vi "SetStringArray.vi"(4 "Sequence Context":T1) -> (0 "error out":errorcluster, 1 "Test Data":T2 {"Numeric Measurement" format="%.2f"})   [LabVIEW 2013]
uses:
  <vilib>/addons/TestStand/_TSLegacy.llb/LabVIEW Test - Test Data.ctl
  <vilib>/addons/TestStand/_TSLegacy.llb/LabVIEW Test - Sequence Context.ctl
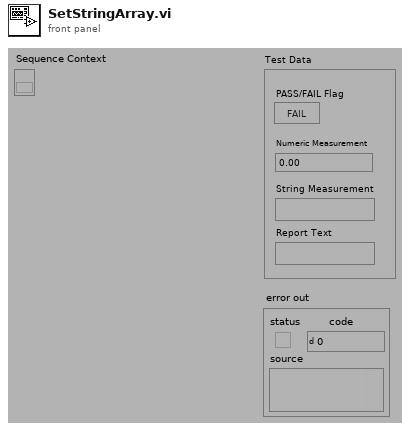
[diagram p1: front panel]
types:
  T1 = typedef "LabVIEW Test - Sequence Context.ctl" = refnum<k7>
  T2 = typedef "LabVIEW Test - Test Data.ctl" = cluster{"PASS/FAIL Flag":bool, "Numeric Measurement":dbl, "String Measurement":string, "Report Text":string}
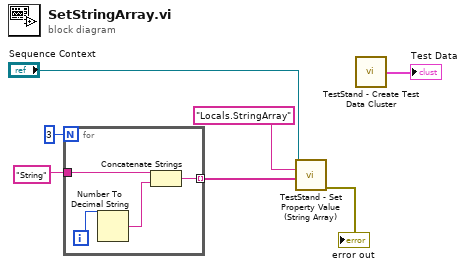
[diagram p0: block diagram]
diagram:
  n1 = for {
    N: 3 -> [_]
    tunnel: "String" -> [w10]
    tunnel: [w8] -> w3 mode=indexing
    i -> [w11]
    n2 = Number To Decimal String(number=w11) -> (decimal integer string=w9:string)  [unwired: 1 out]
    n3 = Concatenate Strings(w10, w9) -> (w8:string)
  }
  n4 = call <vilib>:"TestStand - Set Property Value (String Array).vi"("Sequence Context In"="Sequence Context", "Lookup String"="Locals.StringArray", "New Value"=w3) -> ("error out"=→"error out":errorcluster)  [unwired: 2 in, 10 out]
  n5 = call <vilib>:"TestStand - Create Test Data Cluster.vi"() -> ("Test Data"=→"Test Data":T2)  [unwired: 4 in]
